vi "_Check License.vi"(7 "ApplicationName":string) -> (0 "Reason":string, 1 "Days Left":dbl, 2 "UserName":string, 3 "Valid":bool)   [LabVIEW 2015]
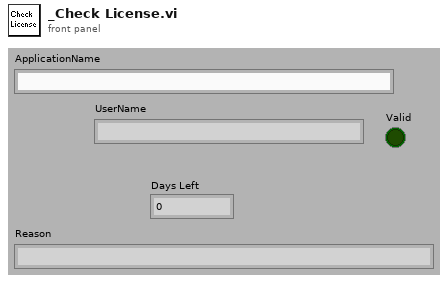
[diagram p1: front panel]
types:
  T1 = cluster{"Company / User Name":string, "Application Name":string, "Version Number (Optional)":string, dbl, dbl, "Key":string}
  T2 = enum16{"open", "replace", "create", "open or create", "replace or create", "replace or create with confirmation"}
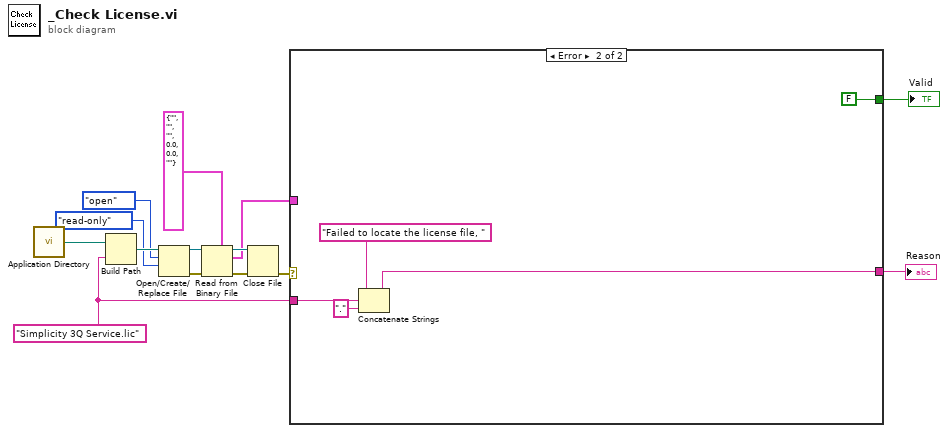
[diagram p0: block diagram]
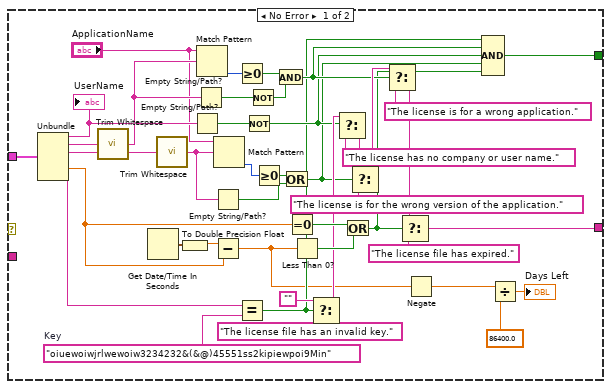
[diagram p2: hidden frame]
diagram:
  w2 = "Simplicity 3Q Service.lic"
  n1 = call <vilib>:"Application Directory.vi"() -> ("Application Directory"=w1:path)
  n2 = Build Path(base path=w1, name or relative path=w2) -> (appended path=w14:path)
  n3 = Open/Create/Replace File(file path (use dialog)=w14, operation (0:open)=T2."open", access (0:read/write)=enum16{"read/write", "read-only", "write-only"}."read-only") -> (refnum out=w11:refnum<file>, error out=w10:errorcluster)  [unwired: 1 in, 3 out]
  n4 = Read from Binary File(5:T1 {"Company / User Name"="", "Application Name"="", "Version Number (Optional)"="", 0.0, 0.0, "Key"=""} ("output cluster"), 8:w10, 11:w11) -> (0:w8:errorcluster, 2:w6:T1, 3:w9:refnum<file>)  [unwired: 4 out]
  n5 = Close File(refnum=w9, error in=w8) -> (error out=w7:errorcluster)  [unwired: 1 out]
  n6 = case shown="Error" w7 {
    tunnel: w6 -> [w57 _]
    tunnel: [w24 FALSE] -> w5
    tunnel: [w23 w58] -> w4
    tunnel: w2 -> [_ w61]
    frame No Error {
      w45 = "oiuewoiwjrlwewoiw3234232&(&@)45551ss2kipiewpoi9Min"  # Key
      n7 = Unbundle(w57) -> ("Company / User Name"=w46:string, "Application Name"=w56:string, "Version Number (Optional)"=w55:string, w17:dbl, "Key"=w22:string)  [unwired: 1 out]
      "UserName" <- w46
      n8 = call <vilib>:"Trim Whitespace.vi"("string"=w56) -> ("trimmed string"=w54:string)  [unwired: 1 in]
      n9 = Get Date/Time In Seconds() -> (seconds since 1Jan1904=w44:timestamp)
      n10 = call <vilib>:"Trim Whitespace.vi"("string"=w55) -> ("trimmed string"=w19:string)  [unwired: 1 in]
      n11 = To Double Precision Float(number=w44) -> (double precision float=w43:dbl)
      n12 = Empty String/Path?(string/path=w46) -> (empty?=w37:bool)
      n13 = Empty String/Path?(string/path=w54) -> (empty?=w51:bool)
      n14 = Match Pattern(string="ApplicationName", regular expression=w54) -> (offset past match=w53:i32)  [unwired: 4 out]
      n15 = Empty String/Path?(string/path=w19) -> (empty?=w47:bool)
      n16 = Subtract(x=w43, y=w17) -> (x-y=w16:dbl)
      n17 = Match Pattern(string="ApplicationName", regular expression=w19) -> (offset past match=w49:i32)  [unwired: 4 out]
      n18 = Greater Or Equal To 0?(x=w53) -> (x >= 0?=w52:bool)
      n19 = Equal?(x=w22, y=w45) -> (x = y?=w25:bool)
      n20 = Not(x=w37) -> (.not. x?=w28:bool)
      n21 = Not(x=w51) -> (.not. x?=w50:bool)
      n22 = Greater Or Equal To 0?(x=w49) -> (x >= 0?=w48:bool)
      n23 = And(x=w52, y=w50) -> (x .and. y?=w29:bool)
      n24 = Or(x=w48, y=w47) -> (x .or. y?=w27:bool)
      n25 = Equal To 0?(x=w17) -> (x = 0?=w42:bool)
      n26 = Less Than 0?(x=w16) -> (x < 0?=w41:bool)
      n27 = Select(t="", s=w25, f="The license file has an invalid key." ("t")) -> (s? t:f=w32:string)
      n28 = Select(t=w32, s=w28, f="The license has no company or user name." ("t")) -> (s? t:f=w33:string)
      n29 = Or(x=w42, y=w41) -> (x .or. y?=w26:bool)
      n30 = Select(t=w33, s=w27, f="The license is for the wrong version of the application." ("t")) -> (s? t:f=w34:string)
      n31 = Select(t=w34, s=w29, f="The license is for a wrong application." ("t")) -> (s? t:f=w35:string)
      n32 = Select(t=w35, s=w26, f="The license file has expired." ("t")) -> (s? t:f=w23:string)
      n33 = Negate(x=w16) -> (-x=w15:dbl)
      n34 = Compound Arithmetic op=AND(w25, w29, w28, w27, w26) -> (w24:bool)
      n35 = Divide(x=w15, y=86400.0) -> (x/y=→"Days Left":dbl)
    }
    frame Error {
      n36 = Concatenate Strings("Failed to locate the license file, ", w61, "." ("string")) -> (w58:string)
    }
  }
  "Valid" <- w5
  "Reason" <- w4
